vi "Stop.vi"(8 "error in (no error)":errorcluster, 11 "EventDaemon in":refnum<class "TemplateDaemon.lvclass">) -> (0 "error out":errorcluster, 3 "EventDaemon out":refnum<class "TemplateDaemon.lvclass">)   [LabVIEW 2024, in "TemplateDaemon.lvclass"]
doc: "Sends stop event to daemon."
uses:
  TemplateDaemon.lvclass
  TemplateDaemon.lvclass/TemplateDaemon.ctl
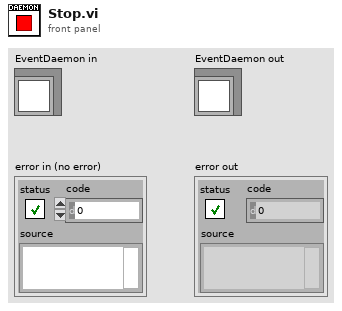
[diagram p1: front panel]
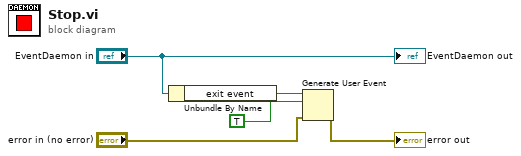
[diagram p0: block diagram]
diagram:
  n1 = Unbundle By Name("EventDaemon in") -> ("exit event"=w5:refnum<user-event>)
  n2 = Generate User Event(user event=w5, event data cluster=TRUE ("event data"), error in="error in (no error)") -> (error out=→"error out":errorcluster)  [unwired: 1 in, 1 out]
  "EventDaemon out" <- "EventDaemon in"
